vi "CODCr通讯.vi"() -> ()   [LabVIEW 2016, in "CODCr库.lvlib"]
uses:
  <vilib>/NI/Modbus Library/API/Wrapper/Create TCP Slave.vi
  <vilib>/NI/Modbus Library/API/slave/Modbus Slave.lvclass
  <vilib>/Plasmionique/MB Master/MB Master.lvlib
  <vilib>/Utility/config.llb/NI_LVConfig.lvlib
  <vilib>/NI/Modbus Library/API/Wrapper/API Main.lvlib
panel:
  out "状态告警区":u16[](array[numeric])
  out "测量数据区":u16[](array[numeric])
  in  "读取参数":bool
  in  "读取数据":bool
  in  "释放串口":bool
  in  "打开串口":bool
  out "队列中元素数量":i32
  out "元素":cluster{"命令":string}[](array[cluster])
  out "待处理插入数量":i32
  out "读取公式":u16[](array[numeric])
  out "读取参数":u16[](array[numeric])
  out "数据存储":u16[](array[numeric])
  out "通讯状态":bool
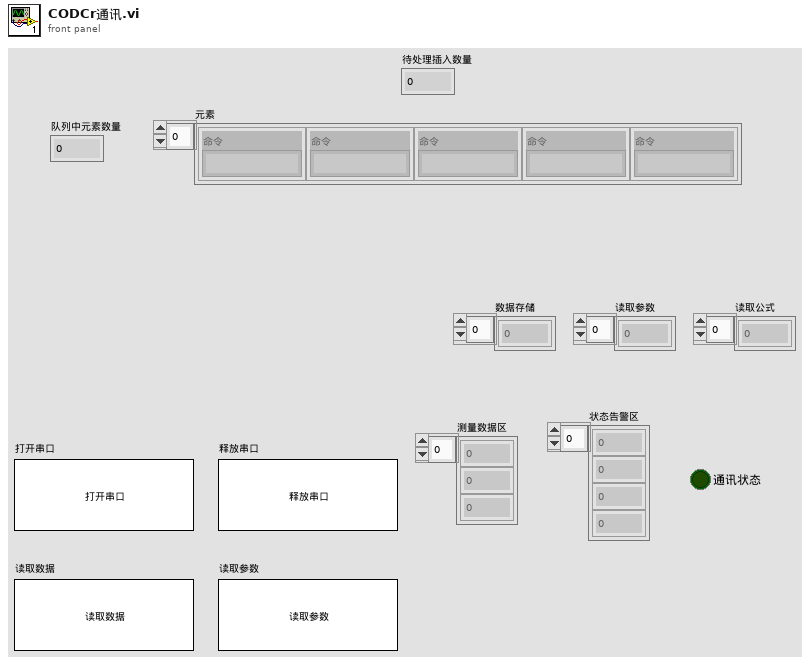
[diagram p1: front panel]
types:
  T1 = typedef "NI_LVConfig.lvlib/Config Data RefNum.ctl" = refnum<k1>
  T2 = cluster{"因子编码":u32, "单位":u16, "标样参考值":sgl, "水样数据时间":timestamp, "水样实测值":sgl, "水样数据标识":string, "标样数据时间":timestamp, "标样实测值":sgl, "标样数据标识":string, "空白数据时间":timestamp, "空白实测值":sgl, "空白数据标识":string, "零点核查数据时间":timestamp, "零点核查实测值":sgl, "零点核查数据标识":string, "跨度核查数据时间":timestamp, "跨度核查实测值":sgl, "跨度核查数据标识":string, "加标回收数据时间":timestamp, "加标回收实测值":sgl, "加标回收数据标识":string, "平行样数据时间":timestamp, "平行样实测值":sgl, "平行样数据标识":string}
  T3 = cluster{"系统时间":timestamp, "工作状态":enum16{"空闲", "水样测试", "标样核查", "零点核查", "跨度核查", "空白测试", "平行样测试", "加标回收", "空白校准", "标样校准", "初始化（清洗）"}, "测量模式":enum16{"待机", "连续模式", "周期模式", "定点模式", "受控模式", "手动模式"}, "告警代码":enum16{"无告警", "缺试剂告警", "缺水样告警", "缺蒸馏水告警", "缺标液告警", "仪表漏液告警", "标定异常告警", "超量程告警", "加热异常", "低试剂预警", "超上限告警", "超下限告警", "仪表内部其他异常", "滴定异常告警", "电极异常告警", "量程切换告警", "参数设置告警", "PH电极电位异常", "电导率电极异常", "浊度光度异常", "溶解氧电极异常", "溶解氧光强异常", "温度异常告警", "PH异常告警", "溶解氧异常告警", "电导率异常告警", "浊度异常告警", "叶绿素异常告警", "藻密度异常告警", "蓝绿藻异常告警", "ORP异常告警", "氨氮异常告警", "清洁刷异常告警", "SD卡异常告警", "蓝牙异常告警", "Wifi异常告警", "流程异常告警"}, "故障代码":enum16{"无故障", "电机故障", "温度故障", "通讯故障", "滴定故障"}, "日志代码":u16, "软件版本":u16, "F0":sgl, "F1":sgl, "F2":sgl, "F3":sgl, "T":sgl, "H":sgl, "id":u16, "flowid":u16, "量程":u16}
  T4 = cluster{"测量精度":u16, "消解温度":u16, "消解时长":u16, "量程下限":sgl, "量程上限":sgl, "曲线斜率K":sgl, "曲线斜率B":sgl, "标定日期":timestamp, "标液1浓度":sgl, "标液1测量过程值":sgl, "标液2浓度":sgl, "标液2测量过程值":sgl, "标液3浓度":sgl, "标液3测量过程值":sgl, "标液4浓度":sgl, "标液4测量过程值":sgl, "标液5浓度":sgl, "标液5测量过程值":sgl, "线性相关系数":sgl, "试剂余量":u32, "测量滴定值或吸光度":sgl, "空白校准时间":timestamp, "标样校准时间":timestamp, "检出限值":sgl, "校准系数":sgl, "设备系列号":string}
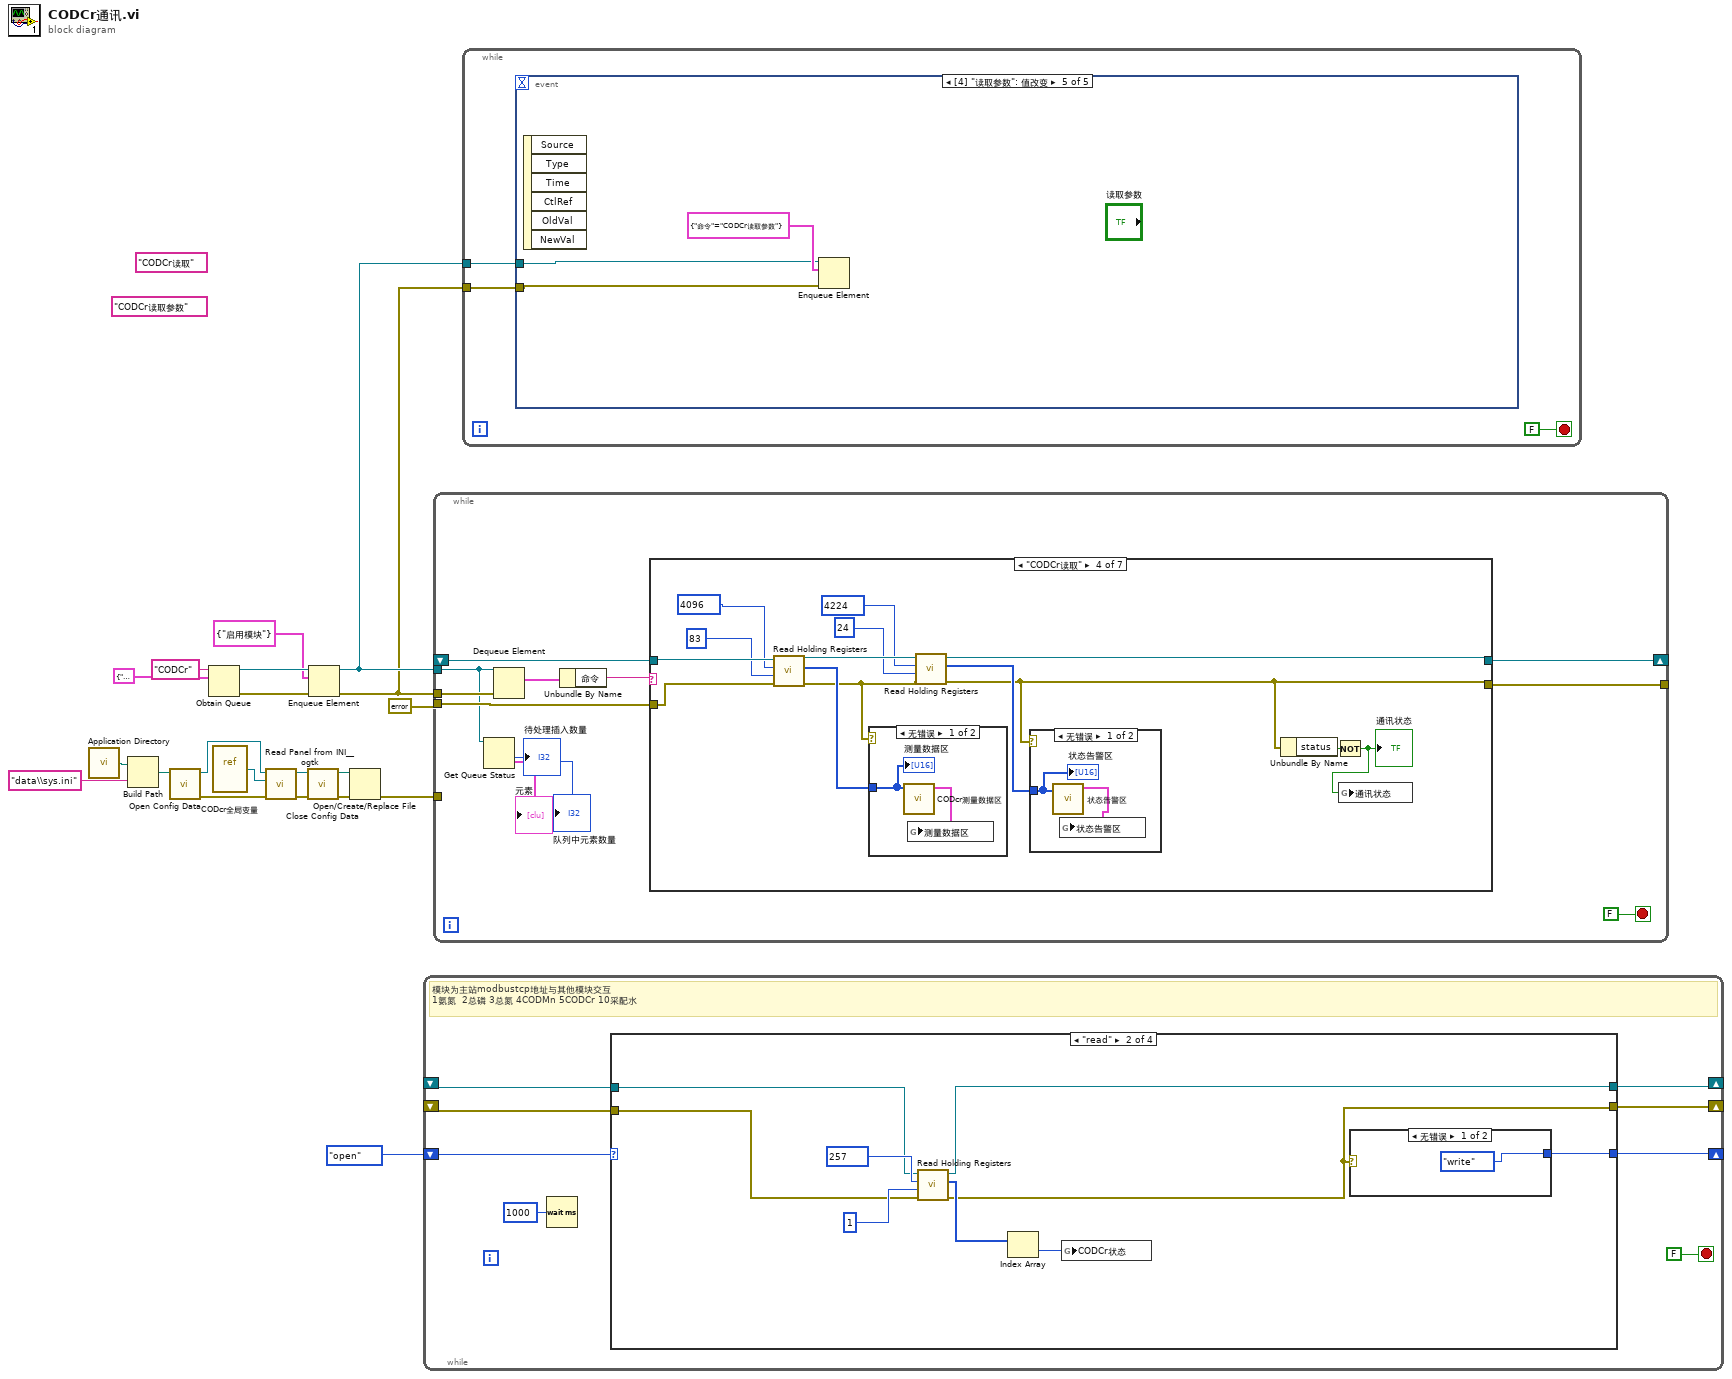
[diagram p0: block diagram]
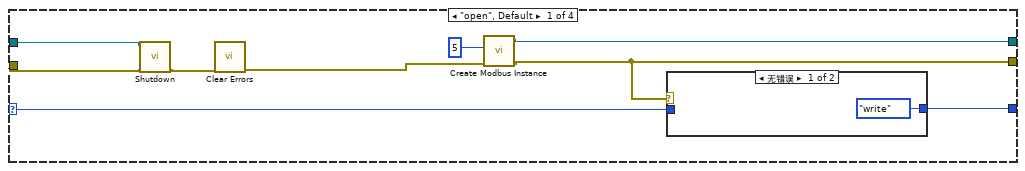
[diagram p2: hidden frame]
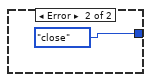
[diagram p4: hidden frame]
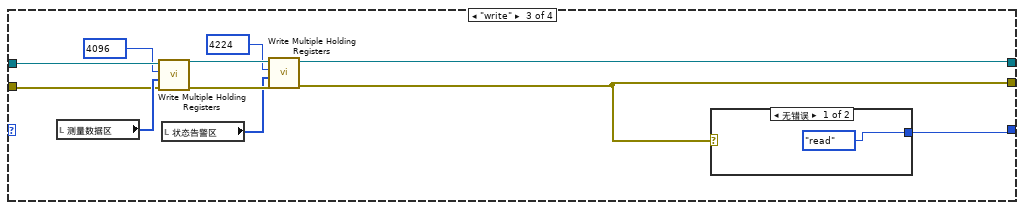
[diagram p5: hidden frame]
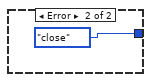
[diagram p6: hidden frame]
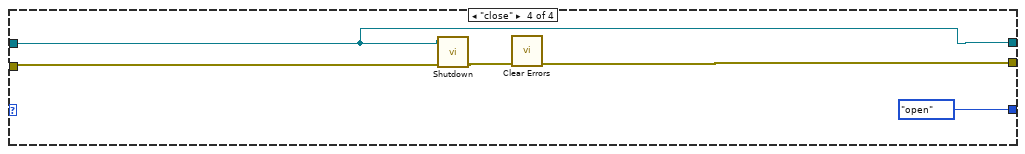
[diagram p7: hidden frame]
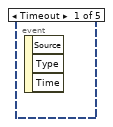
[diagram p8: hidden frame]
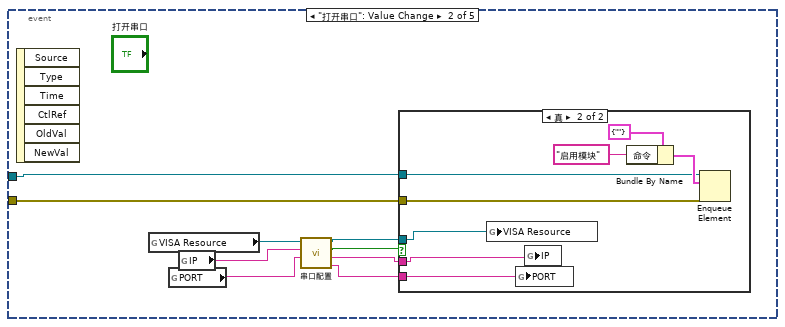
[diagram p9: hidden frame]
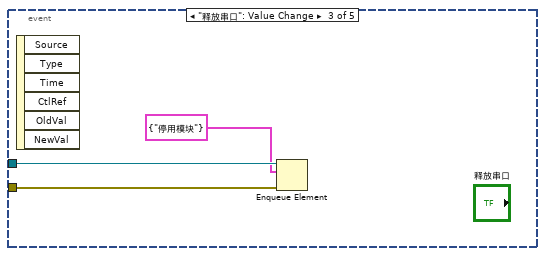
[diagram p11: hidden frame]
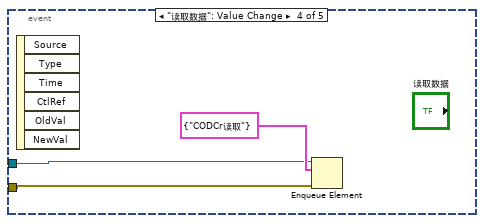
[diagram p12: hidden frame]
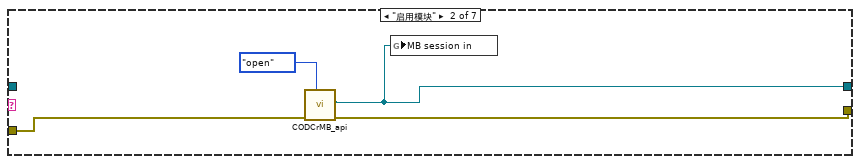
[diagram p14: hidden frame]
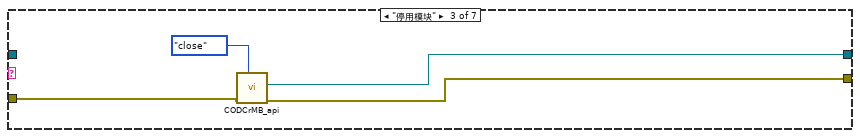
[diagram p15: hidden frame]
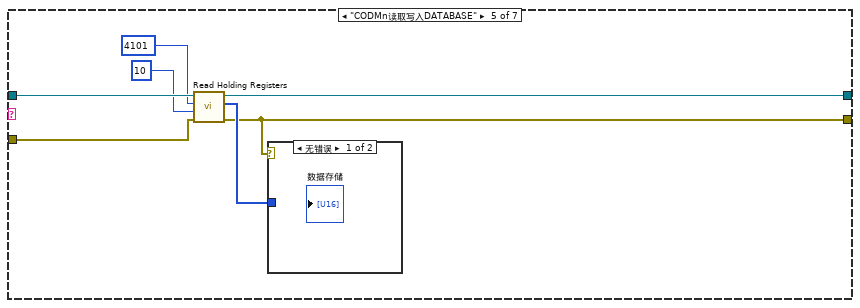
[diagram p18: hidden frame]
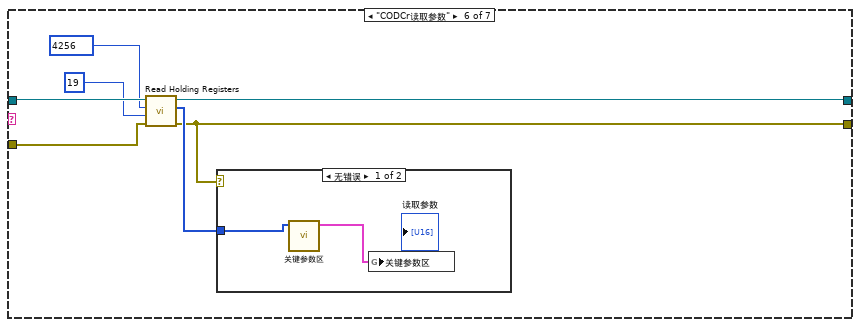
[diagram p20: hidden frame]
diagram:
  (unwired) "CODCr读取参数" ("名称（未命名）")
  (unwired) "CODCr读取" ("名称（未命名）")
  n1 = call <vilib>:"Application Directory.vi"() -> ("Application Directory"=w14:path)
  n2 = Build Path(base path=w14, name or relative path="data\\sys.ini" ("名称或相对路径")) -> (appended path=w12:path)
  n3 = call <vilib>:"Open Config Data.vi"("configuration file path"=w12) -> ("error out"=w8:errorcluster, "refnum"=w11:T1)  [unwired: 8 in, 1 out]
  n4 = Obtain Queue(name (unnamed)="CODCr" ("名称（未命名）"), element data type=cluster{"命令":string} {"命令"="启用模块"} ("元素")) -> (queue out=w17:refnum<queue>, error out=w16:errorcluster)  [unwired: 3 in, 1 out]
  n5 = vi-ref "CODcr全局变量.vi"() -> (w10:refnum<vi>)
  n6 = call <userlib>:"Read Panel from INI__ogtk.vi"("error in (no error)"=w8, "VI ref"=w10, "refnum"=w11) -> ("error out"=w7:errorcluster, "refnum out"=w9:T1)  [unwired: 7 in]
  n7 = call <vilib>:"Close Config Data.vi"("error in (no error)"=w7, "refnum"=w9) -> ("error out"=w6:errorcluster, "file path"=w5:path)  [unwired: 8 in]
  n8 = Enqueue Element(queue=w17, element=cluster{"命令":string} {"命令"="启用模块"} ("元素"), error in (no error)=w16) -> (queue out=w3:refnum<queue>, error out=w2:errorcluster)  [unwired: 1 in, 1 out]
  n9 = Open/Create/Replace File(file path (use dialog)=w5, error in=w6) -> (error out=w4:errorcluster)  [unwired: 4 in, 2 out]
  n10 = while {
    shift-right: [w26] -> _
    shift-left: _ -> [w28]
    shift-right: [w25] -> _
    shift-left: _ -> [w27]
    shift-right: [w22] -> _
    shift-left: enum16{"open", "read", "write", "close"}."open" -> [w23]
    stop <- FALSE stop-if-true
    # "模块为主站modbustcp地址与其他模块交互\n1氨氮  2总磷 3总氮 4CODMn 5CODCr 10采配水"
    n11 = Wait (ms)(milliseconds to wait=u32 1000 ("等待时间（毫秒）")) -> ()  [unwired: 1 out]
    n12 = case shown="\"read\"" w23 {
      selector: w23 -> [w37 _ _ _]
      tunnel: w28 -> [w31 w43 w60 w66]
      tunnel: w27 -> [w30 w42 w56 w65]
      tunnel: [w34 w40 w52 w66] -> w26
      tunnel: [w33 w41 w51 w68] -> w25
      tunnel: [w36 w48 w61 enum16{"open", "read", "write", "close"}."open"] -> w22
      frame "open", Default {
        n13 = call-dynamic "Shutdown.vi"("error in"=w30, "Modbus slave in"=w31) -> ("error out"=w29:errorcluster)  [unwired: 9 in]
        n14 = call <vilib>:"Clear Errors.vi"("error in (no error)"=w29) -> ("error out"=w32:errorcluster)  [unwired: 5 in, 1 out]
        n15 = call-poly <vilib>:"Create Modbus Instance.vi"("error in"=w32, "port (502)"=u16 5) -> ("error out"=w33:errorcluster, "TCP slave instance"=w34:refnum<class "Modbus Slave.lvclass">)  [unwired: 8 in]
        n16 = case shown="无错误" w33 {
          tunnel: w37 -> [_ w39]
          tunnel: [enum16{"open", "read", "write", "close"}."write" w39] -> w36
          frame No Error {
          }
          frame Error {
          }
        }
      }
      frame "read" {
        n17 = call-dynamic <vilib>:"Read Holding Registers.vi"("error in"=w42, "number of inputs"=u16 1, "starting address"=u16 257, "Modbus slave in"=w43) -> ("error out"=w41:errorcluster, "register values"=w45:u16[], "Modbus slave out"=w40:refnum<class "Modbus Slave.lvclass">)  [unwired: 5 in]
        n18 = Index Array(array=w45) -> (element=w44:u16)  [unwired: 1 in]
        n19 = global write "CODCr外部API.vi" "CODCr状态"(w44) -> ()
        n20 = case shown="无错误" w41 {
          tunnel: [enum16{"open", "read", "write", "close"}."write" enum16{"open", "read", "write", "close"}."close"] -> w48
          frame No Error {
          }
          frame Error {
          }
        }
      }
      frame "write" {
        n21 = local read "测量数据区"() -> (w58:u16[])
        n22 = call-dynamic "Write Multiple Holding Registers.vi"("error in"=w56, "registers to write"=w58, "starting address"=u16 4096, "Modbus slave in"=w60) -> ("error out"=w55:errorcluster, "Modbus slave out"=w57:refnum<class "Modbus Slave.lvclass">)  [unwired: 6 in]
        n23 = local read "状态告警区"() -> (w53:u16[])
        n24 = call-dynamic "Write Multiple Holding Registers.vi"("error in"=w55, "registers to write"=w53, "starting address"=u16 4224, "Modbus slave in"=w57) -> ("error out"=w51:errorcluster, "Modbus slave out"=w52:refnum<class "Modbus Slave.lvclass">)  [unwired: 6 in]
        n25 = case shown="无错误" w51 {
          tunnel: [enum16{"open", "read", "write", "close"}."read" enum16{"open", "read", "write", "close"}."close"] -> w61
          frame No Error {
          }
          frame Error {
          }
        }
      }
      frame "close" {
        n26 = call-dynamic "Shutdown.vi"("error in"=w65, "Modbus slave in"=w66) -> ("error out"=w64:errorcluster)  [unwired: 9 in]
        n27 = call <vilib>:"Clear Errors.vi"("error in (no error)"=w64) -> ("error out"=w68:errorcluster)  [unwired: 5 in, 1 out]
      }
    }
  }
  n28 = while {
    tunnel: w3 -> [w72]
    tunnel: w2 -> [w79]
    tunnel: [w73] -> _
    shift-right: [w76] -> _
    shift-left: _ -> [w75]
    tunnel: errorcluster {"status"=FALSE, "code"=0, "source"=""} ("error out") -> [w74]
    tunnel: w4 -> [_]
    stop <- FALSE stop-if-true
    n29 = Get Queue Status(queue=w72) -> (# pending insert=→"待处理插入数量":i32, # elements in queue=→"队列中元素数量":i32, elements=→"元素":cluster{"命令":string}[])  [unwired: 2 in, 5 out]
    n30 = Dequeue Element(queue=w72, error in (no error)=w79) -> (element=w78:cluster{"命令":string})  [unwired: 1 in, 3 out]
    n31 = Unbundle By Name(w78) -> ("命令"=w77:string)
    n32 = case shown="\"CODCr读取\"" w77 {
      tunnel: [w82 w83 w87 w98 w111 w119 w128] -> w76
      tunnel: [w81 w86 w88 w91 w109 w118 w127] -> w73
      tunnel: w75 -> [w82 _ _ w104 w115 w122 w131]
      tunnel: w74 -> [w81 w84 w89 w103 w112 w121 w130]
      frame Default {
      }
      frame "启用模块" {
        n33 = call "CODCrMB_api.vi"("STEP"=enum16{"open", "read", "write", "close"}."open", "Error in"=w84) -> ("error out"=w86:errorcluster, "MB session out"=w83:refnum<class "MB_Master.lvclass">)  [unwired: 7 in, 1 out]
        n34 = global write "CODCr外部API.vi" "MB session in"(w83) -> ()
      }
      frame "停用模块" {
        n35 = call "CODCrMB_api.vi"("STEP"=enum16{"open", "read", "write", "close"}."close", "Error in"=w89) -> ("error out"=w88:errorcluster, "MB session out"=w87:refnum<class "MB_Master.lvclass">)  [unwired: 7 in, 1 out]
      }
      frame "CODCr读取" {
        n36 = call <vilib>:"Read Holding Registers.vi"("error in (no error)"=w103, "quantity"=u16 83 ("number of holding registers"), "starting address"=u16 4096, "MB session in"=w104) -> ("error out"=w100:errorcluster, "Registers"=w102:u16[], "MB session out"=w101:refnum<class "MB_Master.lvclass">)  [unwired: 5 in]
        n37 = case shown="无错误" w100 {
          tunnel: w102 -> [w107 _]
          frame No Error {
            n38 = call "CODcr测量数据区.vi"("数组"=w107) -> ("测量数据区"=w108:T2)  [unwired: 10 in]
            n39 = global write "CODcr全局变量.vi" "测量数据区"(w108) -> ()
            "测量数据区" <- w107
          }
          frame Error {
          }
        }
        n40 = call <vilib>:"Read Holding Registers.vi"("error in (no error)"=w100, "quantity"=u16 24 ("number of holding registers"), "starting address"=u16 4224, "MB session in"=w101) -> ("error out"=w91:errorcluster, "Registers"=w99:u16[], "MB session out"=w98:refnum<class "MB_Master.lvclass">)  [unwired: 5 in]
        n41 = case shown="无错误" w91 {
          tunnel: w99 -> [w105 _]
          frame No Error {
            n42 = call "状态告警区.vi"("数组"=w105) -> ("状态告警区"=w106:T3)  [unwired: 10 in]
            n43 = global write "CODcr全局变量.vi" "状态告警区"(w106) -> ()
            "状态告警区" <- w105
          }
          frame Error {
          }
        }
        n44 = Unbundle By Name(w91) -> ("status"=w92:bool)
        n45 = Not(x=w92) -> (.not. x?=w93:bool)
        "通讯状态" <- w93
        n46 = global write "CODcr全局变量.vi" "通讯状态"(w93) -> ()
      }
      frame "CODMn读取写入DATABASE" {
        n47 = call <vilib>:"Read Holding Registers.vi"("error in (no error)"=w112, "quantity"=u16 10 ("number of holding registers"), "starting address"=u16 4101, "MB session in"=w115) -> ("error out"=w109:errorcluster, "Registers"=w110:u16[], "MB session out"=w111:refnum<class "MB_Master.lvclass">)  [unwired: 5 in]
        n48 = case shown="无错误" w109 {
          tunnel: w110 -> [_ _]
          frame No Error {
          }
          frame Error {
          }
        }
      }
      frame "CODCr读取参数" {
        n49 = call <vilib>:"Read Holding Registers.vi"("error in (no error)"=w121, "quantity"=u16 19 ("number of holding registers"), "starting address"=u16 4256, "MB session in"=w122) -> ("error out"=w118:errorcluster, "Registers"=w120:u16[], "MB session out"=w119:refnum<class "MB_Master.lvclass">)  [unwired: 5 in]
        n50 = case shown="无错误" w118 {
          tunnel: w120 -> [w123 _]
          frame No Error {
            n51 = call "关键参数区.vi"("数组"=w123) -> ("关键参数区"=w124:T4)  [unwired: 10 in]
            n52 = global write "CODcr全局变量.vi" "关键参数区"(w124) -> ()
          }
          frame Error {
          }
        }
      }
      frame "CODMn读取公式" {
        n53 = call <vilib>:"Read Holding Registers.vi"("error in (no error)"=w130, "quantity"=u16 94 ("number of holding registers"), "starting address"=u16 4616, "MB session in"=w131) -> ("error out"=w127:errorcluster, "Registers"=w129:u16[], "MB session out"=w128:refnum<class "MB_Master.lvclass">)  [unwired: 5 in]
        n54 = case shown="无错误" w127 {
          tunnel: w129 -> [_ _]
          frame No Error {
          }
          frame Error {
          }
        }
      }
    }
  }
  n55 = while {
    tunnel: w3 -> [w133]
    tunnel: w2 -> [w132]
    stop <- FALSE stop-if-true
    n56 = event shown="[4] \"读取参数\": 值改变" {
      selector: _ -> [_ _ _ _ _]
      dyn-events: _ -> [_ _ _ _ _]
      timeout: _ -> [_ _ _ _ _]
      tunnel: w133 -> [_ w143 w154 w156 w159]
      tunnel: w132 -> [_ w142 w153 w155 w158]
      event Timeout {
        n57 = event-data() -> ()  [unwired: 1 in, 3 out]
      }
      event "打开串口": Value Change {
        n58 = event-data() -> ()  [unwired: 1 in, 6 out]
        n59 = global read "CODcr全局变量.vi" "VISA Resource"() -> (w141:refnum<visa-resource-name>)
        n60 = global read "CODcr全局变量.vi" "PORT"() -> (w135:string)
        n61 = global read "CODcr全局变量.vi" "IP"() -> (w136:string)
        n62 = call "串口配置.vi"("PORT"=w135, "IP"=w136, "请选择串口:"=w141) -> ("PORT 2"=w137:string, "IP 2"=w138:string, "确认 2"=w140:bool, "VISA资源名称 2"=w139:refnum<visa-resource-name>)  [unwired: 5 in]
        n63 = case shown="真" w140 {
          tunnel: w139 -> [_ w146]
          tunnel: w143 -> [_ w148]
          tunnel: w142 -> [_ w147]
          tunnel: w138 -> [_ w145]
          tunnel: w137 -> [_ w144]
          frame False {
          }
          frame True {
            n64 = global write "CODcr全局变量.vi" "VISA Resource"(w146) -> ()
            n65 = global write "CODcr全局变量.vi" "PORT"(w144) -> ()
            n66 = global write "CODcr全局变量.vi" "IP"(w145) -> ()
            n67 = Bundle By Name(cluster=cluster{"命令":string} {"命令"=""} ("元素"), "命令"="启用模块" ("名称（未命名）")) -> (w149:cluster{"命令":string})
            n68 = Enqueue Element(queue=w148, element=w149, error in (no error)=w147) -> ()  [unwired: 1 in, 3 out]
          }
        }
      }
      event "释放串口": Value Change {
        n69 = event-data() -> ()  [unwired: 1 in, 6 out]
        n70 = Enqueue Element(queue=w154, element=cluster{"命令":string} {"命令"="停用模块"} ("元素"), error in (no error)=w153) -> ()  [unwired: 1 in, 3 out]
      }
      event "读取数据": Value Change {
        n71 = event-data() -> ()  [unwired: 1 in, 6 out]
        n72 = Enqueue Element(queue=w156, element=cluster{"命令":string} {"命令"="CODCr读取"} ("元素"), error in (no error)=w155) -> ()  [unwired: 1 in, 3 out]
      }
      event "读取参数": Value Change {
        n73 = event-data() -> ()  [unwired: 1 in, 6 out]
        n74 = Enqueue Element(queue=w159, element=cluster{"命令":string} {"命令"="CODCr读取参数"} ("元素"), error in (no error)=w158) -> ()  [unwired: 1 in, 3 out]
      }
    }
  }
